vi "Self-Test.vi"(0 "VISA resource name":refnum<visa-resource-name>, 11 "error in (no error)":errorcluster) -> (4 "VISA resource name out":refnum<visa-resource-name>, 6 "Self-Test Result Code":i32, 10 "Self-Test Result Message":string, 15 "error out":errorcluster)   [LabVIEW 2016, in "APT 300XAC Series.lvlib"]
doc: "Performs a self test of the instrument data memory. Returns 0 if it is successful or 1 if the test fails."
uses:
  APT 300XAC Series.lvlib
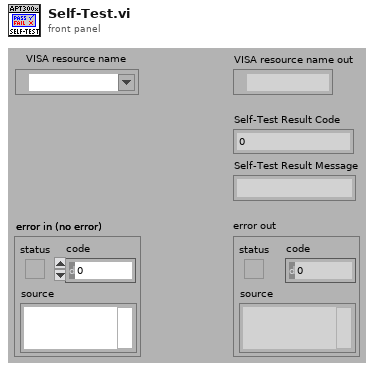
[diagram p1: front panel]
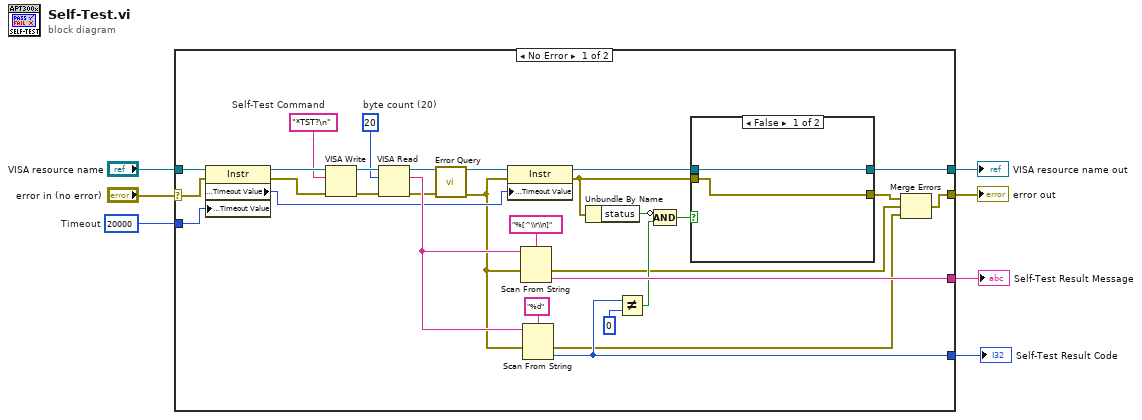
[diagram p0: block diagram]
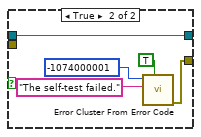
[diagram p2: hidden frame]
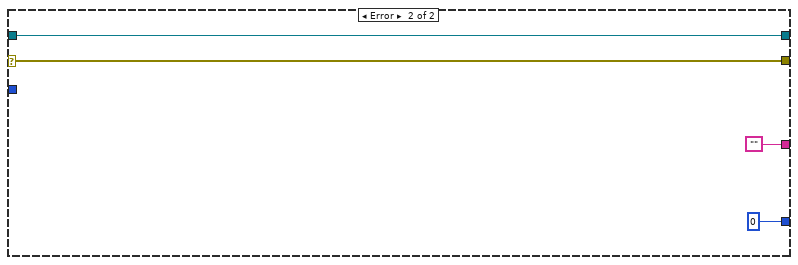
[diagram p3: hidden frame]
diagram:
  w3 = u32 20000  # Timeout
  n1 = case shown="No Error" "error in (no error)" {
    selector: "error in (no error)" -> [w17 w47]
    tunnel: "VISA resource name" -> [w33 w48]
    tunnel: [w12 w48] -> w6
    tunnel: [w13 w47] -> w5
    tunnel: [w30 "" ("Empty String Constant")] -> w4
    tunnel: w3 -> [w29 _]
    tunnel: [w19 0] -> w2
    frame No Error {
      w32 = u32 20  # byte count (20)
      w25 = "*TST?\n"  # Self-Test Command
      n2 = property on="Property Node" class="Instr"(reference=w33, error in=w17, "General Settings:Timeout Value"=w29) -> (reference out=w27:refnum<visa-resource-name>, error out=w28:errorcluster, "General Settings:Timeout Value"=w26:u32)
      n3 = VISA Write(VISA resource name=w27, write buffer=w25, error in (no error)=w28) -> (VISA resource name out=w35:refnum<visa-resource-name>, error out=w34:errorcluster)  [unwired: 1 out]
      n4 = VISA Read(VISA resource name=w35, byte count=w32, error in (no error)=w34) -> (VISA resource name out=w11:refnum<visa-resource-name>, read buffer=w31:string, error out=w10:errorcluster)  [unwired: 1 out]
      n5 = call "Error Query.vi"("VISA resource name"=w11, "error in (no error)"=w10) -> ("VISA resource name out"=w9:refnum<visa-resource-name>, "error out"=w8:errorcluster)  [unwired: 10 in, 2 out]
      n6 = property on="Property Node" class="Instr"(reference=w9, error in=w8, "General Settings:Timeout Value"=w26) -> (reference out=w24:refnum<visa-resource-name>, error out=w23:errorcluster)
      n7 = Scan From String(format string="%[^\\r\\n]" ("Format String"), input string=w31, error in=w8) -> (error out=w14:errorcluster, output 1=w30:string)  [unwired: 2 in, 2 out]
      n8 = Scan From String(format string="%d", input string=w31, error in=w8) -> (error out=w15:errorcluster, output 1=w19:i32)  [unwired: 2 in, 2 out]
      n9 = Unbundle By Name(w23) -> ("status"=w21:bool)
      n10 = Not Equal?(x=w19, y=0) -> (x != y?=w22:bool)
      n11 = Compound Arithmetic op=AND(invert w21, w22) -> (w20:bool)
      n12 = case shown="False" w20 {
        tunnel: w24 -> [w39 w44]
        tunnel: w23 -> [w38 _]
        tunnel: [w38 w40] -> w16
        tunnel: [w39 w44] -> w12
        frame False {
        }
        frame True {
          n13 = call <vilib>:"Error Cluster From Error Code.vi"("show call chain? (False)"=TRUE, "error message (\"\")"="The self-test failed." ("Source (VI Name)"), "error code (0)"=-1074000001 ("Code")) -> ("error out"=w40:errorcluster)  [unwired: 6 in]
        }
      }
      n14 = Merge Errors(w16, w14, w15) -> (w13:errorcluster)
    }
    frame Error {
    }
  }
  "Self-Test Result Message" <- w4
  "Self-Test Result Code" <- w2
  "VISA resource name out" <- w6
  "error out" <- w5
